vi "CSV_Setup_Data_Handler.vi"(0 "first iteration":bool, 1 "Timeout 1":bool, 7 "Sample Data":dbl[](array[numeric]), 9 "Sample Data 2":dbl[](array[numeric]), 11 "Data":T1={"system"={"info"={"menuSelect"=0, "version"=0, "serial"="", "captureActive"=FALSE, "captureBegin"=FALSE, "emptyAndRefill"=FALSE}, "userInfo"={"operatorName"="", "date"=timestamp(2713993200 s since 1904-01-01)}, "camera"={"exposureTime"=0, "aperture"=enum."Item 0", "framerate"=0, "framerateMax"=0, "legacyAttributes"=FALSE}}, "connections"={"arduino"={"connection"="", "status"=FALSE, "openState"=FALSE, "emptyStart"=0}, "pump"={"connection"="", "status"=FALSE, "command"="", "dispenseSpeed"=100, "flushSize"=100}, "camera"={"cam1"={"connection"="", "status"=FALSE}, "cam2"={"connection"="", "status"=FALSE}}}, "queue"={"process"={"cam1"=refnum, "cam2"=refnum, "queueSize"=0}, "save"={"cam1"=refnum, "cam2"=refnum, "queueSize"=0}, "overloadThreshold"=0}, "imageProcess"={"cam1"={"preAllocation"={"image"="Station", "originalDisplay"="Station", "originalRgb"="Station", "binary"="Station", "save"="Station", "calibrationFull"=refnum, "calibrationDetect"=refnum}, "calibration"={"pathFull"=path "", "pathDetect"=path "", "ROI"={"Left"=0, "Top"=0, "Right"=0, "Bottom"=0, "Rotation"=0.0}}}, "cam2"={"preAllocation"={"image"=refnum, "originalDisplay"=refnum, "originalRgb"=refnum, "binary"=refnum, "save"=refnum, "calibrationFull"=refnum, "calibrationDetect"=refnum}, "calibration"={"pathFull"=path "", "pathDetect"=path "", "ROI"={"Left"=0, "Top"=0, "Right"=0, "Bottom"=0, "Rotation"=0.0}}}, "process"={"planeExtract"=refnum, "planeSubtract"=refnum, "cropMask"=refnum}, "detection"={"sampleTimeout"=0, "sizeThreshold"=0, "detectionRegionPct"=0.0}}, "sampleData"={"sampleId"="", "projectId"="", "voucherID"="", "speciesName"="", "collectionDate"=timestamp(2713993200 s since 1904-01-01), "sampleStation"="", "location"="", "lat"=0.0, "lon"=0.0, "determiner"="", "sex"="", "otherNotes"=""}, "Session In"=""} {"sampleData"."collectionDate" format="%<%Y-%m-%d>T"; "imageProcess"."detection"."sizeThreshold" min=1; "imageProcess"."cam2"."calibration"."ROI"."Rotation" format="%.2f"; "imageProcess"."cam2"."calibration"."ROI"."Left" scale=0.0..1024.0; "imageProcess"."cam2"."calibration"."ROI"."Right" scale=0.0..1024.0; "imageProcess"."cam1"."calibration"."ROI"."Rotation" format="%.2f"; "imageProcess"."cam1"."calibration"."ROI"."Left" scale=0.0..1024.0; "imageProcess"."cam1"."calibration"."ROI"."Right" scale=0.0..1024.0; "queue"."overloadThreshold" min=1; "queue"."save"."queueSize" min=1; "queue"."process"."queueSize" min=1; "connections"."pump"."flushSize" min=1; "connections"."pump"."dispenseSpeed" min=1; "system"."camera"."framerateMax" min=1; "system"."userInfo"."date" format="%<%Y-%m-%dT%H:%M:%S+%z>T"; "system"."info"."version" items=["Standard", "XL"]; "system"."info"."menuSelect" items=["Session Data", "Extended Setup", "Buffer", "Camera", "Dispenser", "Stats", "Connections"]}, 12 "Timeout 2":bool) -> (4 "Sample Name":string, 10 "Cam1_Stats":cluster{"Mean_Area":i32, "Img_Count":u32} caption="Camera 1", 15 "Cam2_Stats":cluster{"Mean_Area":i32, "Img_Count":u32} caption="Camera 2")   [LabVIEW 2022 SP3]
uses:
  controls/Data.ctl
  <vilib>/userdefined/High Color/IMAQdx.ctl
  <vilib>/vision/Image Controls.llb/IMAQ Image.ctl
panel:
  in  "Stop":bool
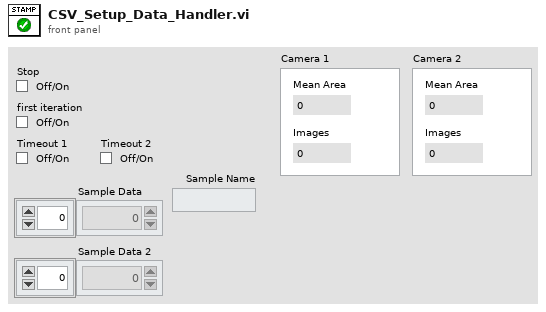
[diagram p1: front panel]
types:
  T1 = typedef "Data.ctl" = cluster{"system":cluster{"info":cluster{"menuSelect":u16, "version":u16, "serial":string, "captureActive":bool, "captureBegin":bool, "emptyAndRefill":bool}, "userInfo":cluster{"operatorName":string, "date":timestamp}, "camera":cluster{"exposureTime":i32, "aperture":enum32{"Item 0", "Item 1", "Item 2", "Item 3"}, "framerate":i32, "framerateMax":i32, "legacyAttributes":bool}}, "connections":cluster{"arduino":cluster{"connection":refnum<visa-resource-name>, "status":bool, "openState":bool, "emptyStart":u32}, "pump":cluster{"connection":refnum<visa-resource-name>, "status":bool, "command":string, "dispenseSpeed":i32, "flushSize":i32}, "camera":cluster{"cam1":cluster{"connection":T2, "status":bool}, "cam2":cluster{"connection":T2, "status":bool}}}, "queue":cluster{"process":cluster{"cam1":refnum<queue>, "cam2":refnum<queue>, "queueSize":i32}, "save":cluster{"cam1":refnum<queue>, "cam2":refnum<queue>, "queueSize":i32}, "overloadThreshold":i32}, "imageProcess":cluster{"cam1":cluster{"preAllocation":cluster{"image":T3, "originalDisplay":T3, "originalRgb":T3, "binary":T3, "save":T3, "calibrationFull":T3, "calibrationDetect":T3}, "calibration":cluster{"pathFull":path, "pathDetect":path, "ROI":T4}}, "cam2":cluster{"preAllocation":cluster{"image":T3, "originalDisplay":T3, "originalRgb":T3, "binary":T3, "save":T3, "calibrationFull":T3, "calibrationDetect":T3}, "calibration":cluster{"pathFull":path, "pathDetect":path, "ROI":T4}}, "process":cluster{"planeExtract":T3, "planeSubtract":T3, "cropMask":T3}, "detection":cluster{"sampleTimeout":i32, "sizeThreshold":i32, "detectionRegionPct":dbl}}, "sampleData":cluster{"sampleId":string, "projectId":string, "voucherID":string, "speciesName":string, "collectionDate":timestamp, "sampleStation":string, "location":string, "lat":dbl, "lon":dbl, "determiner":string, "sex":string, "otherNotes":string}, "Session In":T2}
  T2 = typedef "IMAQdx.ctl" = refnum<k21>
  T3 = typedef "IMAQ Image.ctl" = refnum<image>
  T4 = typedef "IMAQ Rectangle" = cluster{"Left":i32, "Top":i32, "Right":i32, "Bottom":i32, "Rotation":dbl}
  T5 = cluster{"MFD max":string, "MFD mean":string, "MFD std. dev.":string, "Perim. mean":string, "Perim. std. dev":string, "Area mean":string, "Area std. dev.":string, "Holes mean":string, "Holes std. dev.":string, "Area+Holes mean":string, "Area+Holes std. dev.":string, "numberOfImages":string}
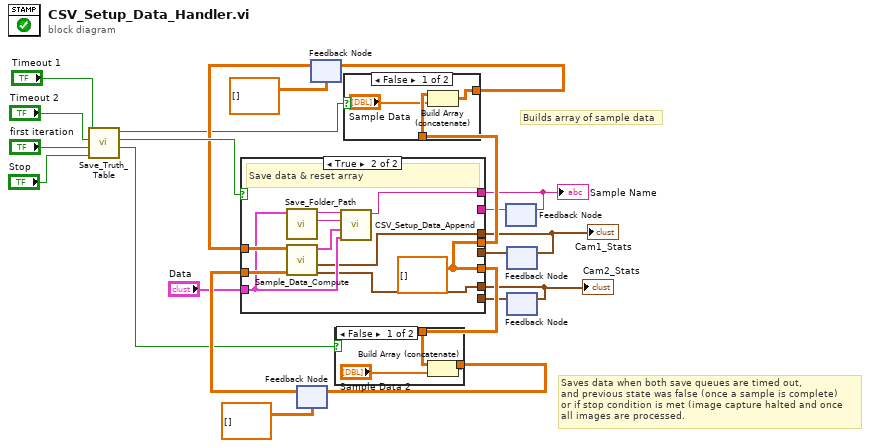
[diagram p0: block diagram]
diagram:
  # "Builds array of sample data"
  # "Saves data when both save queues are timed out, \nand previous state was false (once a sample is complete)\nor if stop condition is met (image capture halted and once\nall images are processed."
  n1 = call "Save_Truth_Table.vi"("Stop"="Stop", "first iteration"="first iteration", "Timeout 2"="Timeout 2", "Timeout 1"="Timeout 1") -> ("Append Sample Data 2"=w12:bool, "Save_Data"=w15:bool, "Append Sample Data 1"=w13:bool)  [unwired: 5 in]
  n2 = feedback #1(dbl[][] []) -> (w18:dbl[][])
  n3 = feedback #2(dbl[][] []) -> (w14:dbl[][])
  n4 = feedback #3() -> (w5:string)  [unwired: 1 in]
  n5 = feedback #4() -> (w4:cluster{"Mean_Area":i32, "Img_Count":u32})  [unwired: 1 in]
  n6 = feedback #5() -> (w3:cluster{"Mean_Area":i32, "Img_Count":u32})  [unwired: 1 in]
  n7 = case shown="True" w15 {
    tunnel: "Data" -> [_ w33]
    tunnel: w18 -> [w27 w35]
    tunnel: [w27 w36] -> w16
    tunnel: w14 -> [w26 w34]
    tunnel: [w26 w36] -> w22
    tunnel: [w25 w30] -> w6
    tunnel: [w23 w29] -> w2
    tunnel: [w24 w28] -> w1
    tunnel: w5 -> [w25 _]
    tunnel: w4 -> [w24 _]
    tunnel: w3 -> [w23 _]
    frame False {
      # "Build sample array"
    }
    frame True {
      w36 = dbl[][] []
      # "Save data & reset array"
      n8 = call "Save_Folder_Path.vi"("input cluster"=w33) -> ("Subfolder Name"=w32:string, "Subfolder Path"=w31:string)  [unwired: 9 in]
      n9 = call "Sample_Data_Compute.vi"("Data Array 2"=w35, "Data Array 1"=w34) -> ("Cam2_Stats"=w29:cluster{"Mean_Area":i32, "Img_Count":u32}, "Cam1_Stats"=w28:cluster{"Mean_Area":i32, "Img_Count":u32}, "summaryData"=w37:T5)  [unwired: 7 in]
      n10 = call "CSV_Setup_Data_Append.vi"("input cluster"=w33, "summaryData"=w37, "Sample Name"=w32, "Image path"=w31) -> ("Sample Name dup."=w30:string)  [unwired: 7 in]
    }
  }
  "Sample Name" <- w6
  "Cam1_Stats" <- w1
  "Cam2_Stats" <- w2
  n11 = case shown="False" w12 {
    tunnel: [w40 w41] -> w17
    tunnel: w16 -> [w39 w41]
    frame False {
      n12 = Build Array (concatenate)(w39, "Sample Data 2") -> (w40:dbl[][])
    }
    frame True {
    }
  }
  n13 = feedback-in #1(w17) -> ()
  n14 = case shown="False" w13 {
    tunnel: w22 -> [w44 w45]
    tunnel: [w43 w45] -> w19
    frame False {
      n15 = Build Array (concatenate)(w44, "Sample Data") -> (w43:dbl[][])
    }
    frame True {
    }
  }
  n16 = feedback-in #2(w19) -> ()
  n17 = feedback-in #3(w6) -> ()
  n18 = feedback-in #4(w1) -> ()
  n19 = feedback-in #5(w2) -> ()
